vi "Event Loop.vi"(8 "error in (no error)":errorcluster) -> (0 "error out":errorcluster)   [LabVIEW 2020]
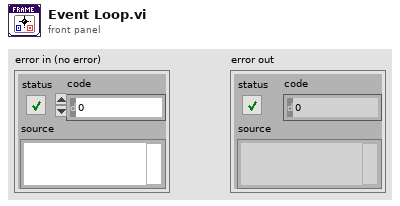
[diagram p1: front panel]
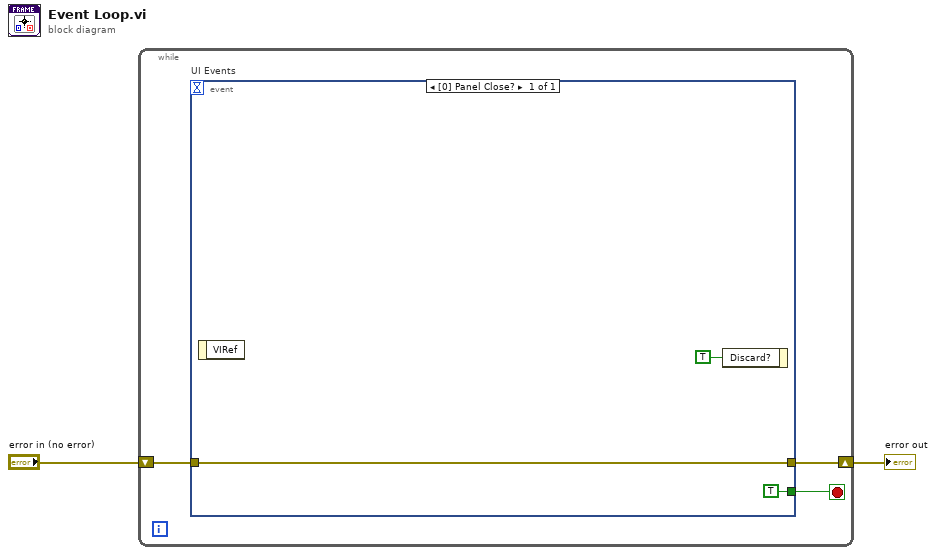
[diagram p0: block diagram]
diagram:
  n1 = while {
    shift-right: [w3] -> w1
    shift-left: "error in (no error)" -> [w4]
    stop <- w5 stop-if-true
    n2 = event "UI Events" shown="[0] Panel Close?" {
      selector: _ -> [_]
      dyn-events: _ -> [_]
      timeout: _ -> [_]
      tunnel: [TRUE ("stop")] -> w5
      tunnel: w4 -> [w7]
      tunnel: [w7] -> w3
      event Panel Close? {
        n3 = event-data() -> ()  [unwired: 1 in, 1 out]
        n4 = event-data("Discard?"=TRUE) -> ()  [unwired: 1 in, 1 out]
      }
    }
  }
  "error out" <- w1
